vi "get child configuration objects.vi"(8 "error in":errorcluster, 10 "serializable node":refnum<class "NISE_CEF_serializable node.lvclass">, 11 "NISE_CEF_HierarchyRepo in":refnum<class "NISE_CEF_HierarchyRepo.lvclass">) -> (0 "error out":errorcluster, 1 "children":refnum<class "NISE_CEF_serializable configuration.lvclass">[](array[class]), 3 "NISE_CEF_HierarchyRepo out":refnum<class "NISE_CEF_HierarchyRepo.lvclass">)   [LabVIEW 2013, in "NISE_CEF_HierarchyRepo.lvclass"]
uses:
  NISE_CEF_HierarchyRepo.lvclass
  serializable node/NISE_CEF_serializable node.lvclass
  serializable configuration/NISE_CEF_serializable configuration.lvclass
  NISE_CEF_HierarchyRepo.lvclass/NISE_CEF_HierarchyRepo.ctl
  serializable configuration/NISE_CEF_serializable configuration.lvclass/NISE_CEF_serializable configuration.ctl
  tree based serializer/NISE_CEF_TreeSerializer.lvlib
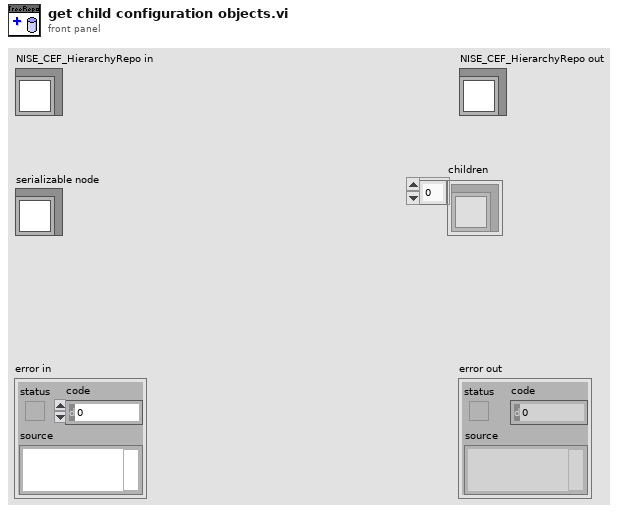
[diagram p1: front panel]
types:
  T1 = typedef "NISE_CEF_TreeSerializer.lvlib/memory hierarchy.ctl" = cluster{"hierarchy":T2[], "instance data":refnum<class "NISE_CEF_serializable configuration.lvclass">[], "root nodes":string[]}
  T2 = typedef "NISE_CEF_TreeSerializer.lvlib/hierarchy element.ctl" = cluster{"current node":string, "children":string[]}
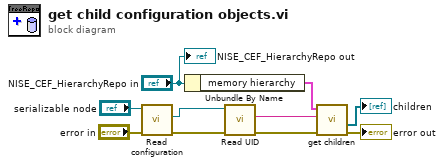
[diagram p0: block diagram]
diagram:
  n1 = call "Read configuration.vi"("error in"="error in", "NISE_CEF_serializable node in"="serializable node") -> ("error out"=w6:errorcluster, "configuration"=w4:refnum<class "NISE_CEF_serializable configuration.lvclass">)  [unwired: 7 in, 1 out]
  n2 = Unbundle By Name("NISE_CEF_HierarchyRepo in") -> ("memory hierarchy"=w7:T1)
  n3 = call "Read UID.vi"("error in"=w6, "configuration in"=w4) -> ("error out"=w5:errorcluster, "instance id"=w3:string)  [unwired: 7 in, 1 out]
  n4 = call "get children.vi"("error in"=w5, "ID"=w3, "memory hierarchy"=w7) -> ("error out"=→"error out":errorcluster, "children"=→"children":refnum<class "NISE_CEF_serializable configuration.lvclass">[])  [unwired: 7 in]
  "NISE_CEF_HierarchyRepo out" <- "NISE_CEF_HierarchyRepo in"
